vi "CSM Module.vi"(11 "CSM Basic Refs":T1) -> (2 "Enum":T2, 3 "CSM Basic Refs (dup)":T1)   [LabVIEW 2017]
uses:
  CSM Basic Refs.ctl
  CSM Module Type.ctl
panel:
  out "Error out":errorcluster
  in  "Error in":errorcluster caption="Error in (no error)"
  out "result":bool
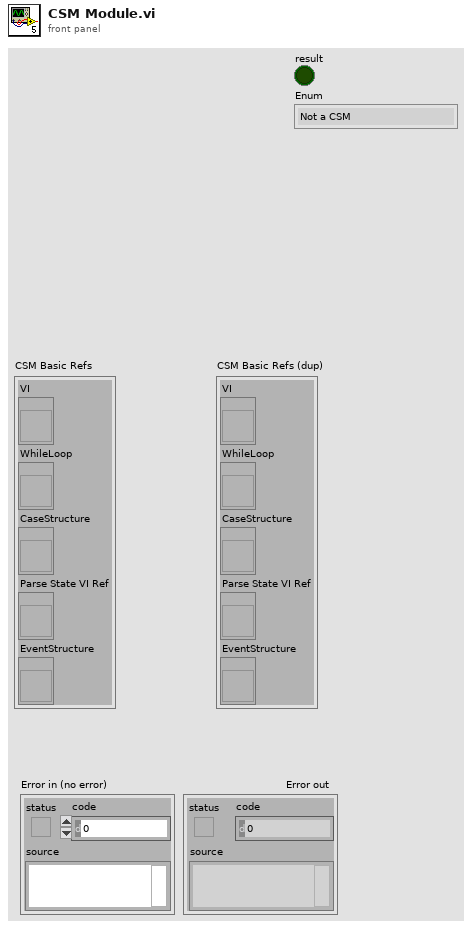
[diagram p1: front panel]
types:
  T1 = typedef "CSM Basic Refs.ctl" = cluster{"VI":refnum<vi>, "WhileLoop":refnum<vi>, "CaseStructure":refnum<vi>, "Parse State VI Ref":refnum<vi>, "EventStructure":refnum<vi>}
  T2 = typedef "CSM Module Type.ctl" = enum16{"Not a CSM", "JKISM", "CSM"}
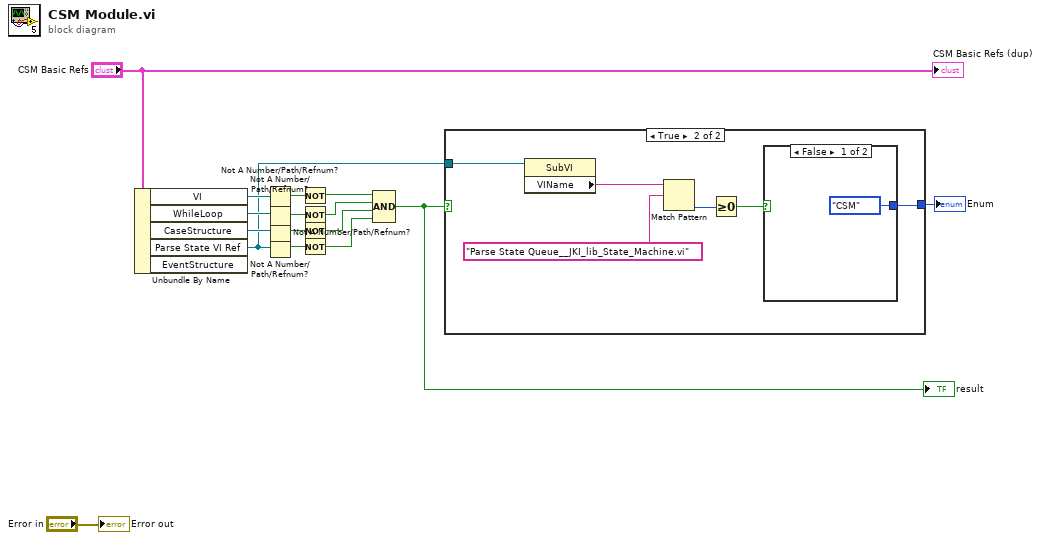
[diagram p0: block diagram]
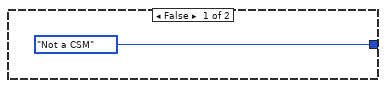
[diagram p2: hidden frame]
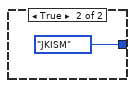
[diagram p3: hidden frame]
diagram:
  n1 = Unbundle By Name("CSM Basic Refs") -> ("VI"=w14:refnum<vi>, "WhileLoop"=w13:refnum<vi>, "CaseStructure"=w11:refnum<vi>, "Parse State VI Ref"=w3:refnum<vi>)  [unwired: 1 out]
  n2 = Not A Number/Path/Refnum?(number/path/refnum=w14) -> (NaN/Path/Refnum?=w16:bool)
  n3 = Not A Number/Path/Refnum?(number/path/refnum=w13) -> (NaN/Path/Refnum?=w15:bool)
  n4 = Not A Number/Path/Refnum?(number/path/refnum=w11) -> (NaN/Path/Refnum?=w12:bool)
  n5 = Not A Number/Path/Refnum?(number/path/refnum=w3) -> (NaN/Path/Refnum?=w10:bool)
  n6 = Not(x=w16) -> (.not. x?=w9:bool)
  n7 = Not(x=w15) -> (.not. x?=w8:bool)
  n8 = Not(x=w12) -> (.not. x?=w7:bool)
  n9 = Not(x=w10) -> (.not. x?=w6:bool)
  n10 = Compound Arithmetic op=AND(w9, w8, w7, w6) -> (w5:bool)
  "result" <- w5
  n11 = case shown="True" w5 {
    tunnel: [CSM_Module_Type."Not a CSM" w23] -> w4
    tunnel: w3 -> [_ w22]
    frame False {
    }
    frame True {
      n12 = property class="SubVI"(reference=w22) -> ("VIName"=w21:string)  [unwired: 1 in, 2 out]
      n13 = Match Pattern(string=w21, regular expression="Parse State Queue__JKI_lib_State_Machine.vi") -> (offset past match=w19:i32)  [unwired: 1 in, 3 out]
      n14 = Greater Or Equal To 0?(x=w19) -> (x >= 0?=w18:bool)
      n15 = case shown="False" w18 {
        tunnel: [CSM_Module_Type."CSM" CSM_Module_Type."JKISM"] -> w23
        frame False {
        }
        frame True {
        }
      }
    }
  }
  "Enum" <- w4
  "CSM Basic Refs (dup)" <- "CSM Basic Refs"
  "Error out" <- "Error in"
